vi "vision process ball.vi"(8 "?":errorcluster, 11 "Processed Image":T1(plugin-control)) -> (2 "Annotated Image Out":T1(plugin-control), 3 "Processed Image Out":T1(plugin-control))   [LabVIEW 2015]
uses:
  <vilib>/vision/NI_Vision_Development_Module.lvlib
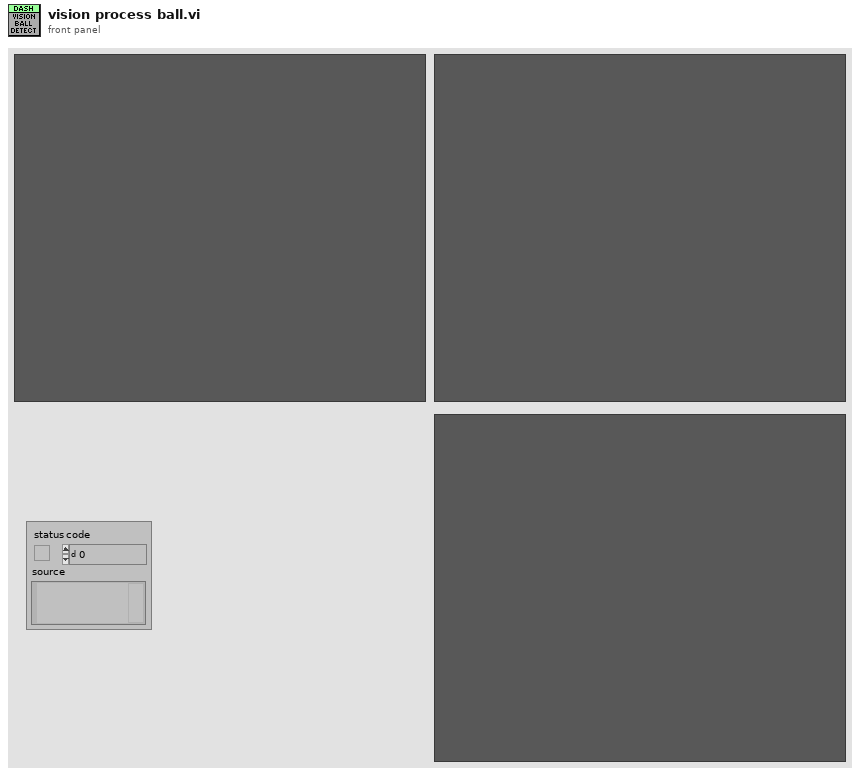
[diagram p1: front panel]
types:
  T1 = typedef "IMAQ Image.ctl" = refnum<image>
  T2 = cluster{"Pos. X":i32, "Pos. Y":i32, "Radius":i32, "Core Area":i32}[]
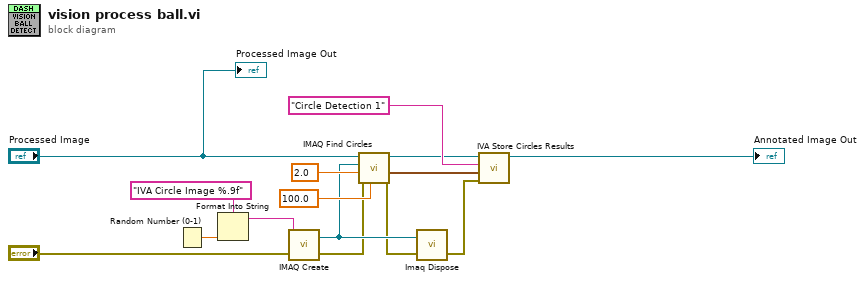
[diagram p0: block diagram]
diagram:
  n1 = Random Number (0-1)() -> (number: 0 to 1=w4:dbl)
  n2 = Format Into String(format string="IVA Circle Image %.9f" ("Image Name"), w4) -> (resulting string=w6:string)  [unwired: 2 in, 1 out]
  n3 = call "IMAQ Create"("Image Name"=w6, "error in (no error)"="?") -> ("New Image"=w12:T1, "error out"=w11:errorcluster)  [unwired: 2 in, 1 out]
  n4 = call "IMAQ Find Circles"("Max Radius"=sgl 100.0, "error in (no error)"=w11, "Min Radius"=sgl 2.0, "Image Dst"=w12, "Image Src"="Processed Image") -> ("error out"=w10:errorcluster, "Circles Data"=w7:T2)  [unwired: 5 out]
  n5 = call "Imaq Dispose"("Image"=w12, "error in (no error)"=w10) -> ("error out"=w9:errorcluster)  [unwired: 1 in, 3 out]
  n6 = call <vilib>:"IVA Store Circles Results.vi"("error in (no error)"=w9, "Circles Data"=w7, "Step Name"="Circle Detection 1", "Image in"="Processed Image") -> ("Image dup"=→"Annotated Image Out":T1)  [unwired: 7 out]
  "Processed Image Out" <- "Processed Image"
